vi "禹山电导率校准.vi"() -> ()   [LabVIEW 2016, in "斯坦道多参数.lvlib"]
uses:
  <vilib>/Utility/miscctls.llb/LVPointTypeDef.ctl
  <vilib>/Analysis/NI_AALBase.lvlib
  <vilib>/Analysis/NI_AALPro.lvlib
panel:
  out "滤波设定":dbl
  out "盐度":dbl caption="盐度测量值" format="%#.2f"
  out "通讯状态":string
  out "第二点校准值":dbl
  out "第一点校准值":dbl
  out "最小值":sgl format="%.2g"
  out "最大值":sgl format="%.2g"
  in  "校准停止":bool
  in  "校准模式":u16(ring) items=["两点校准", "单点校准"]
  in  "标液2":dbl
  in  "标液1":dbl
  out "波形图表":sgl(graph) caption="历史曲线"
  out "温度测量值":dbl caption="温度" format="%#.2f"
  out "变异系数":dbl format="%.6g"
  out "standard deviation":dbl caption="标准差" format="%0.2f"
  out "mean":dbl caption="均值" format="%0.2f"
  out "提示":string
  in  "校准启动":bool
  out "测试值":dbl format="%#.2f"
  out "电极斜率":dbl format="%#.6f"
  out "电极零点":dbl format="%#.6f"
  # "电导率电极设定"
  # "℃"
  # "μS/cm"
  # "ppt"
  # "请选择校准模式:"
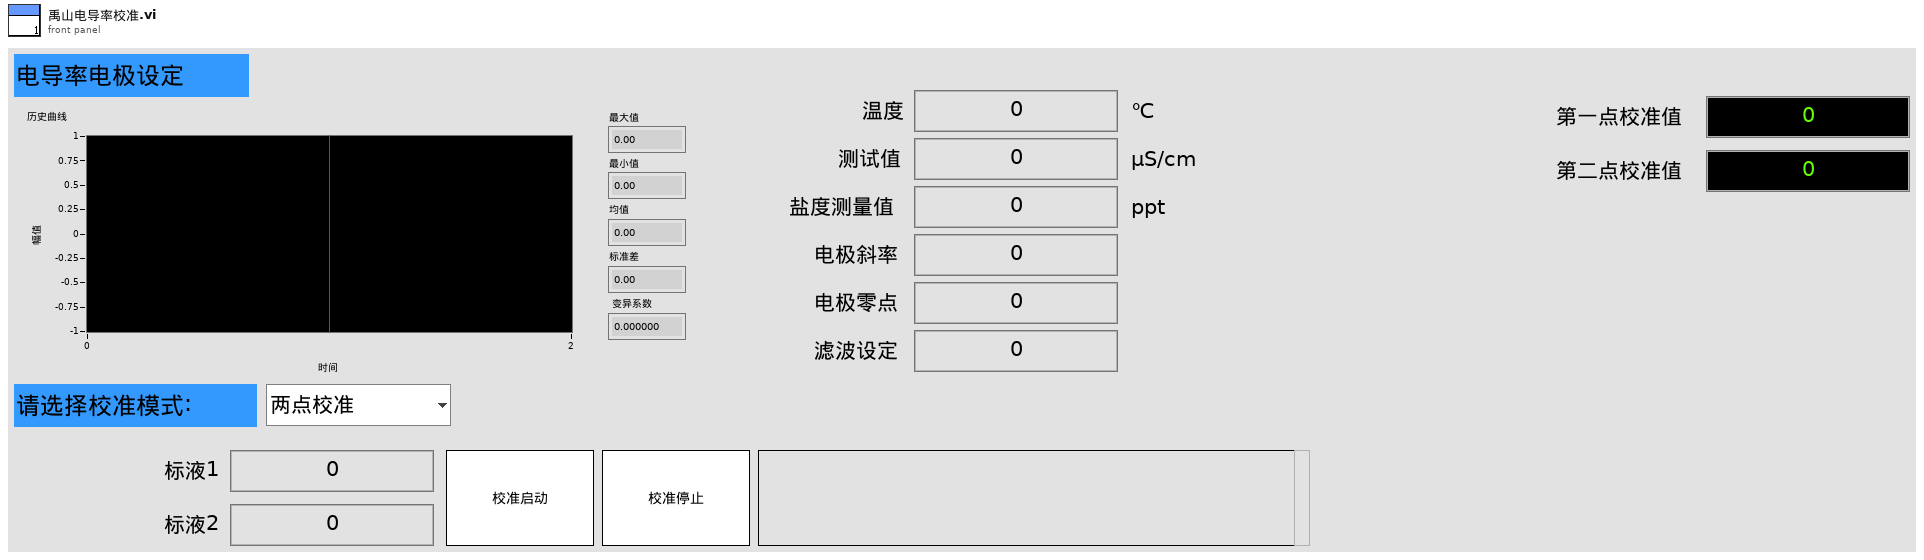
[diagram p1: front panel]
types:
  T1 = typedef "斯坦道多参数.lvlib/通知队列类型.ctl" = enum16{"pH", "DO", "DO2", "Cond", "Turb", "ORP", "叶绿素a", "藻密度", "COD"}
  T2 = typedef "LVPointTypeDef.ctl" = cluster{"Horizontal":i16, "Vertical":i16}
  T3 = cluster{"pH":u32, "DO":u32, "Cond":u32, "Turb":u32, "叶绿素a":u32, "藻密度":u32, "ORP":u32, "COD":u32}
  T4 = cluster{"温度测量值":sgl, "测量值":sgl, "温度偏移修正值":sgl, "信号值":sgl, "数据标识":string}
  T5 = enum8{"Enabled", "Disabled", "Disabled and Grayed Out"}
  T6 = cluster{"ph":bool, "DO":bool, "Cond":bool, "Turb":bool, "叶绿素a":bool, "藻密度":bool, "ORP":bool, "COD":bool, "DO2":bool}
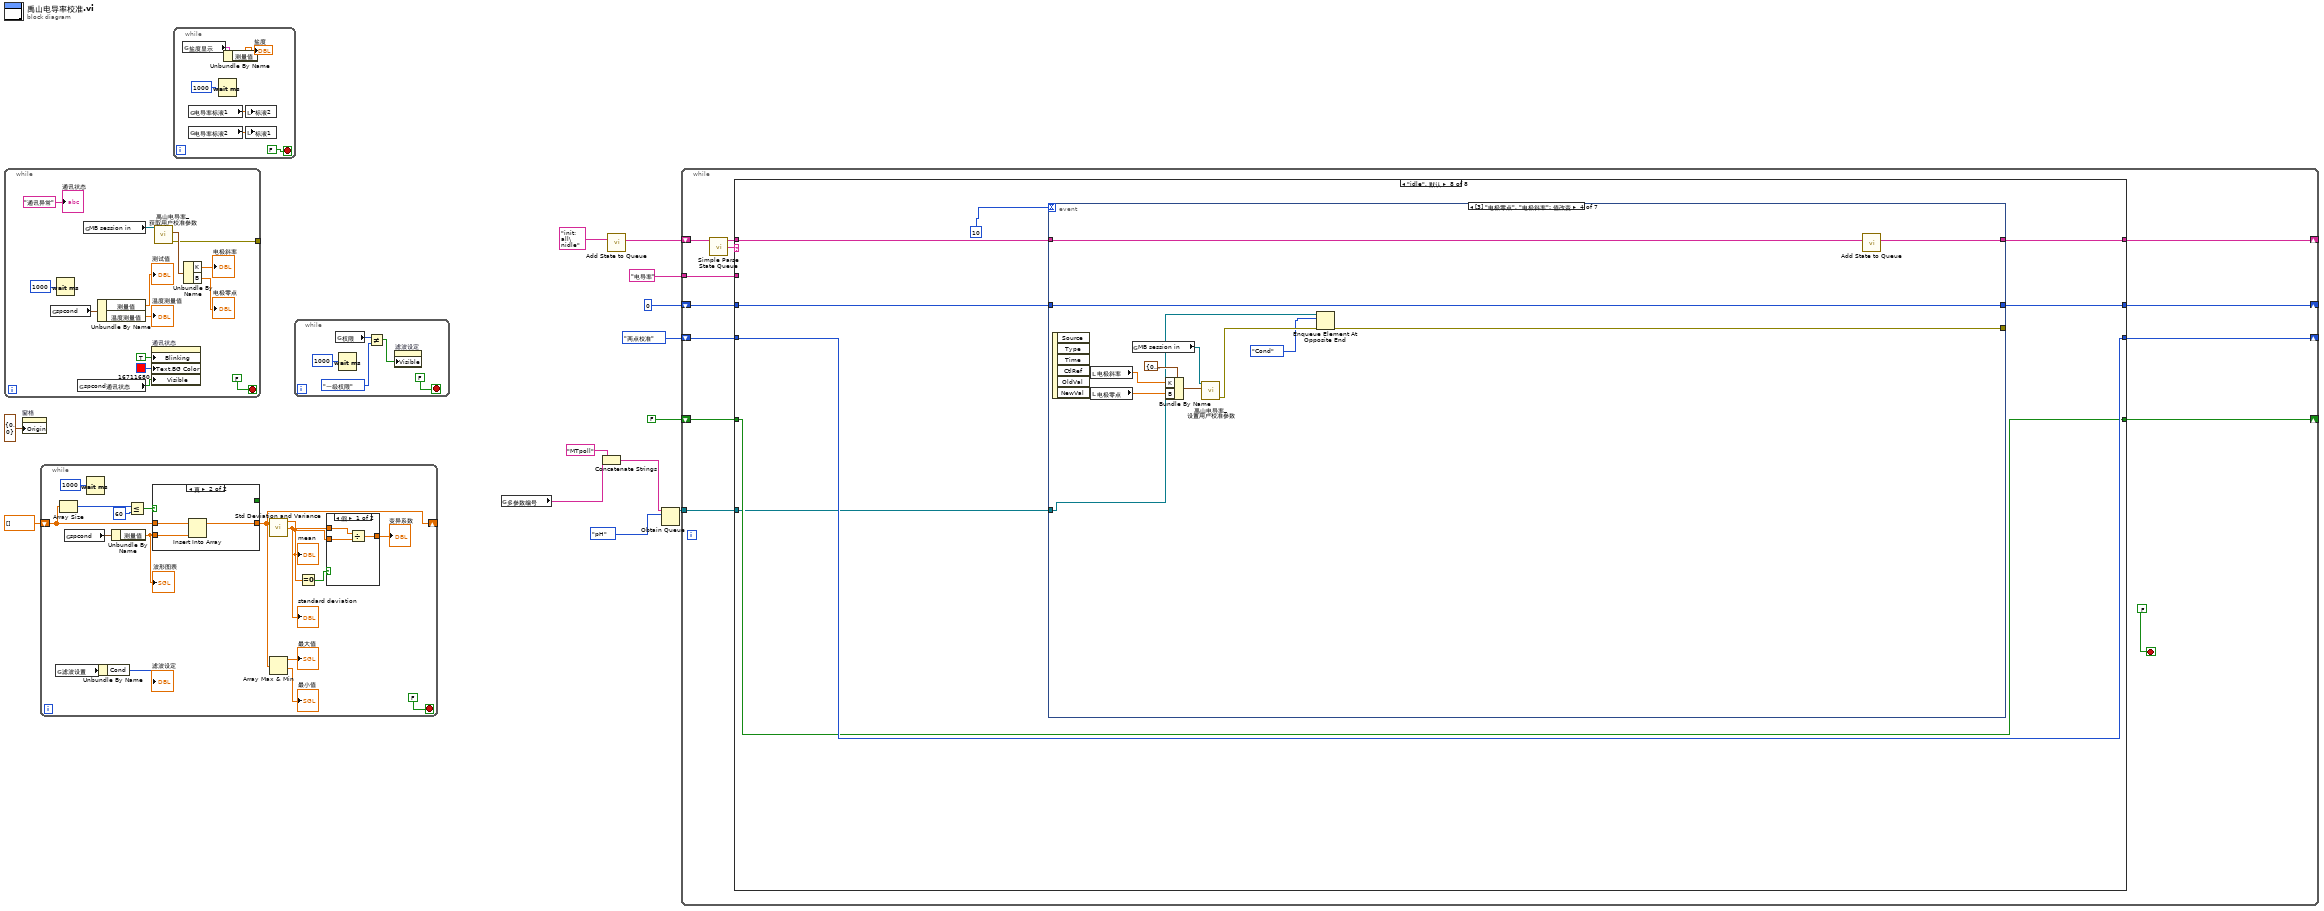
[diagram p0: block diagram]
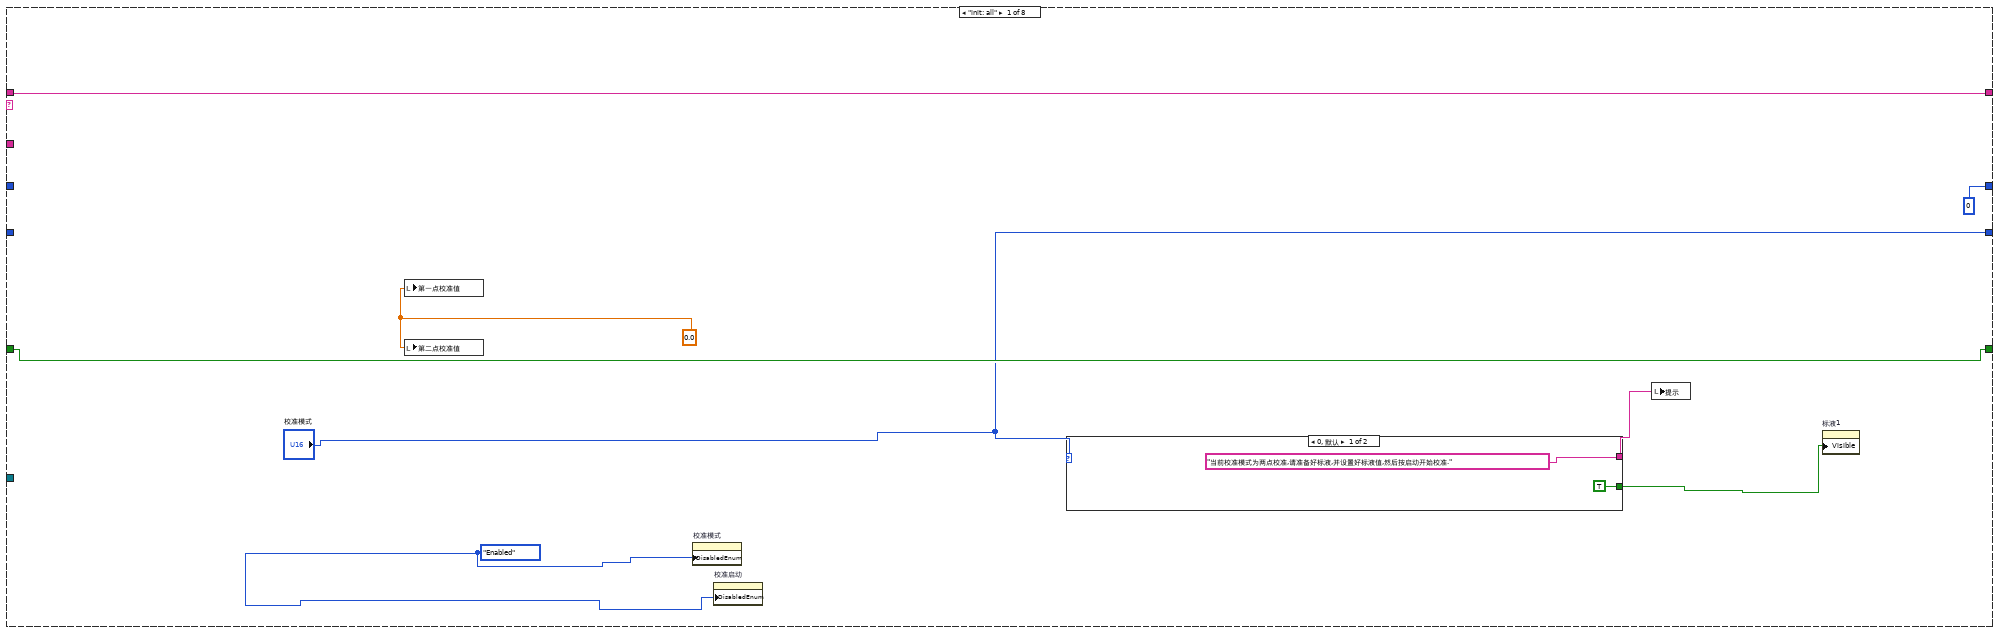
[diagram p2: hidden frame]
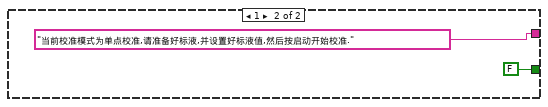
[diagram p3: hidden frame]
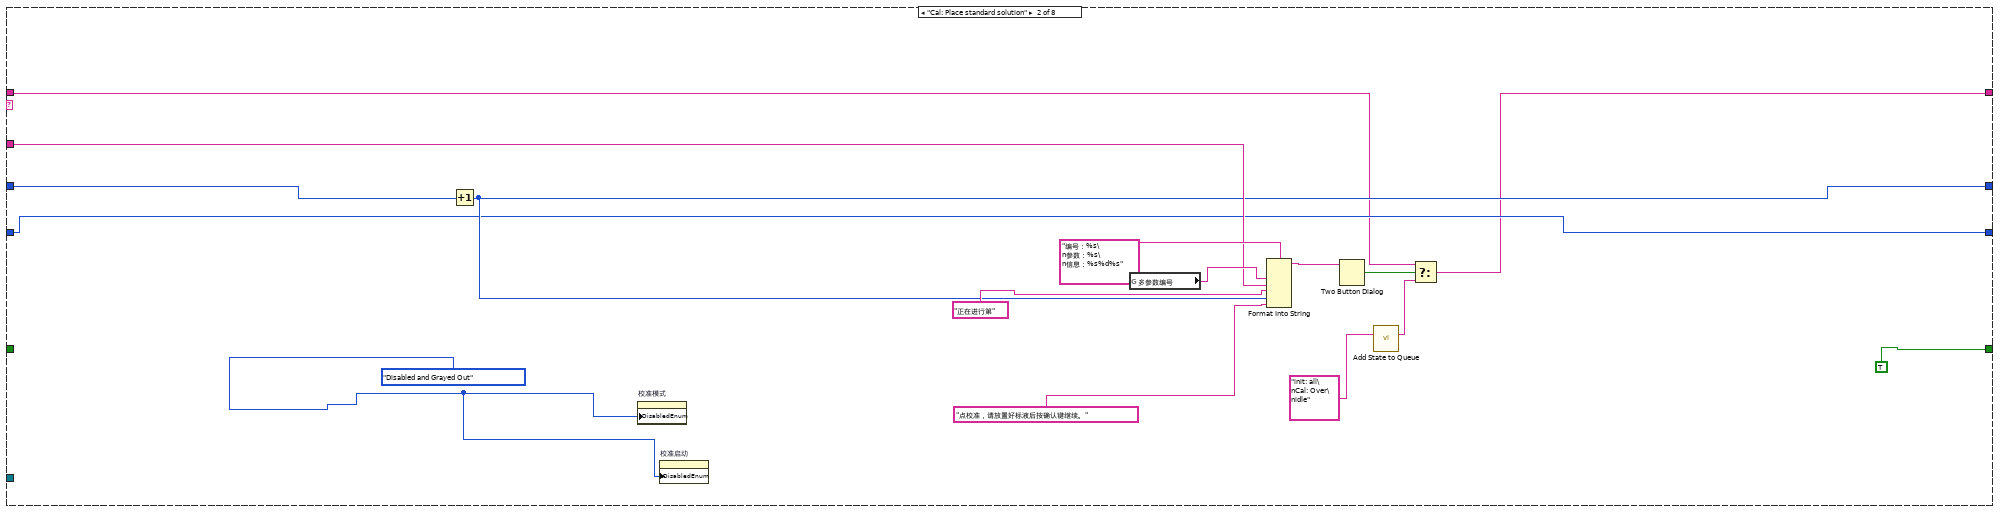
[diagram p4: hidden frame]
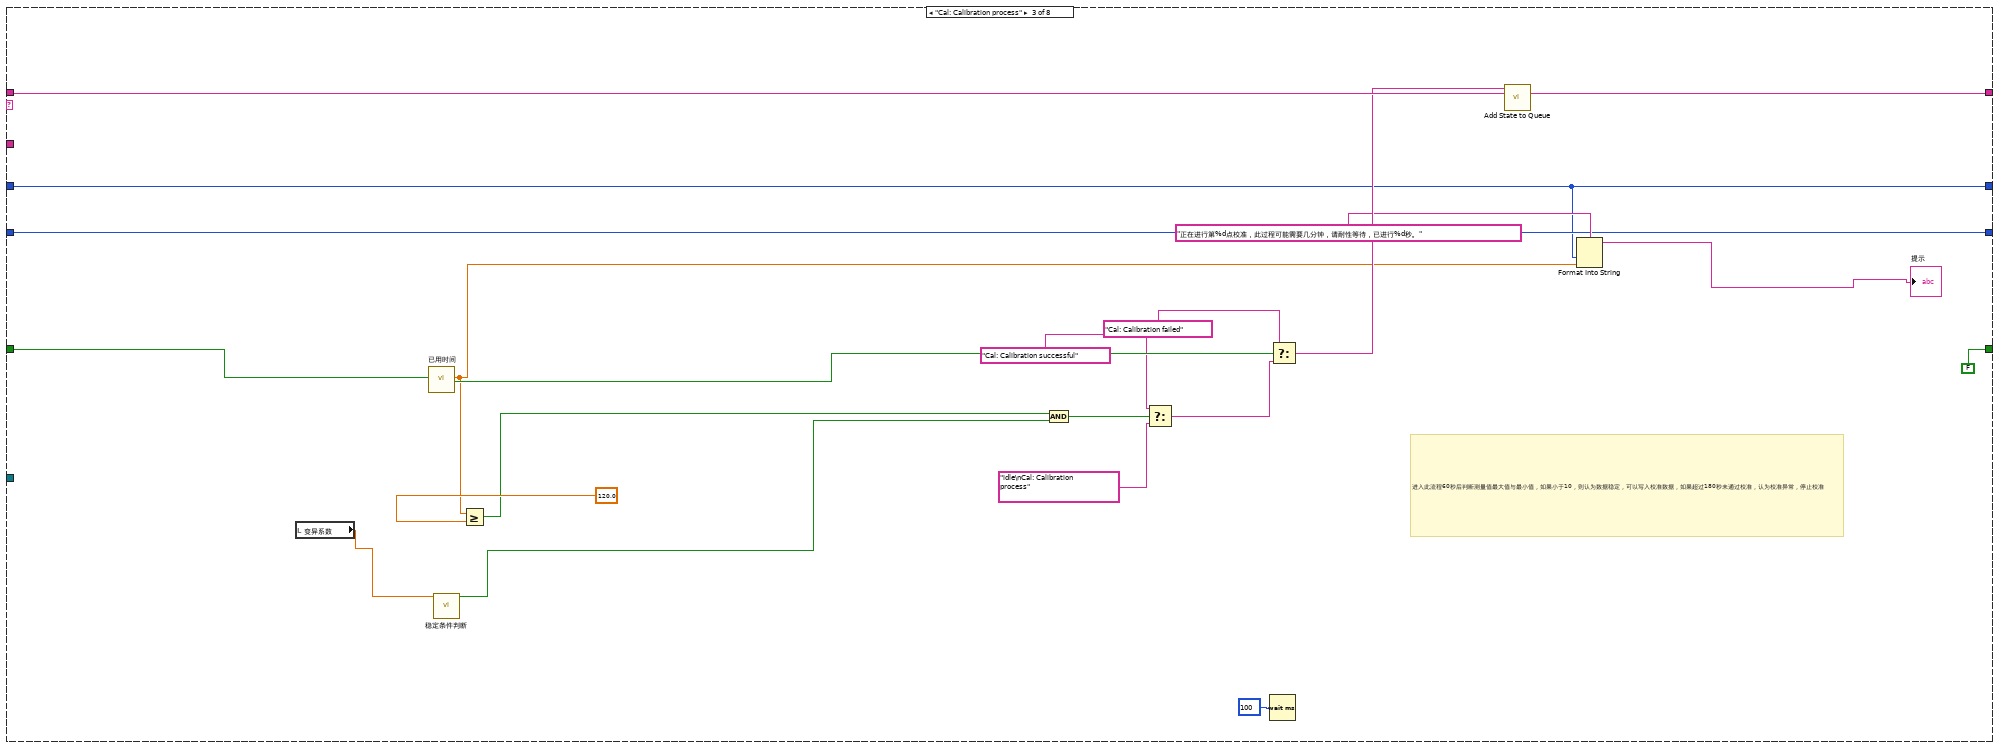
[diagram p5: hidden frame]
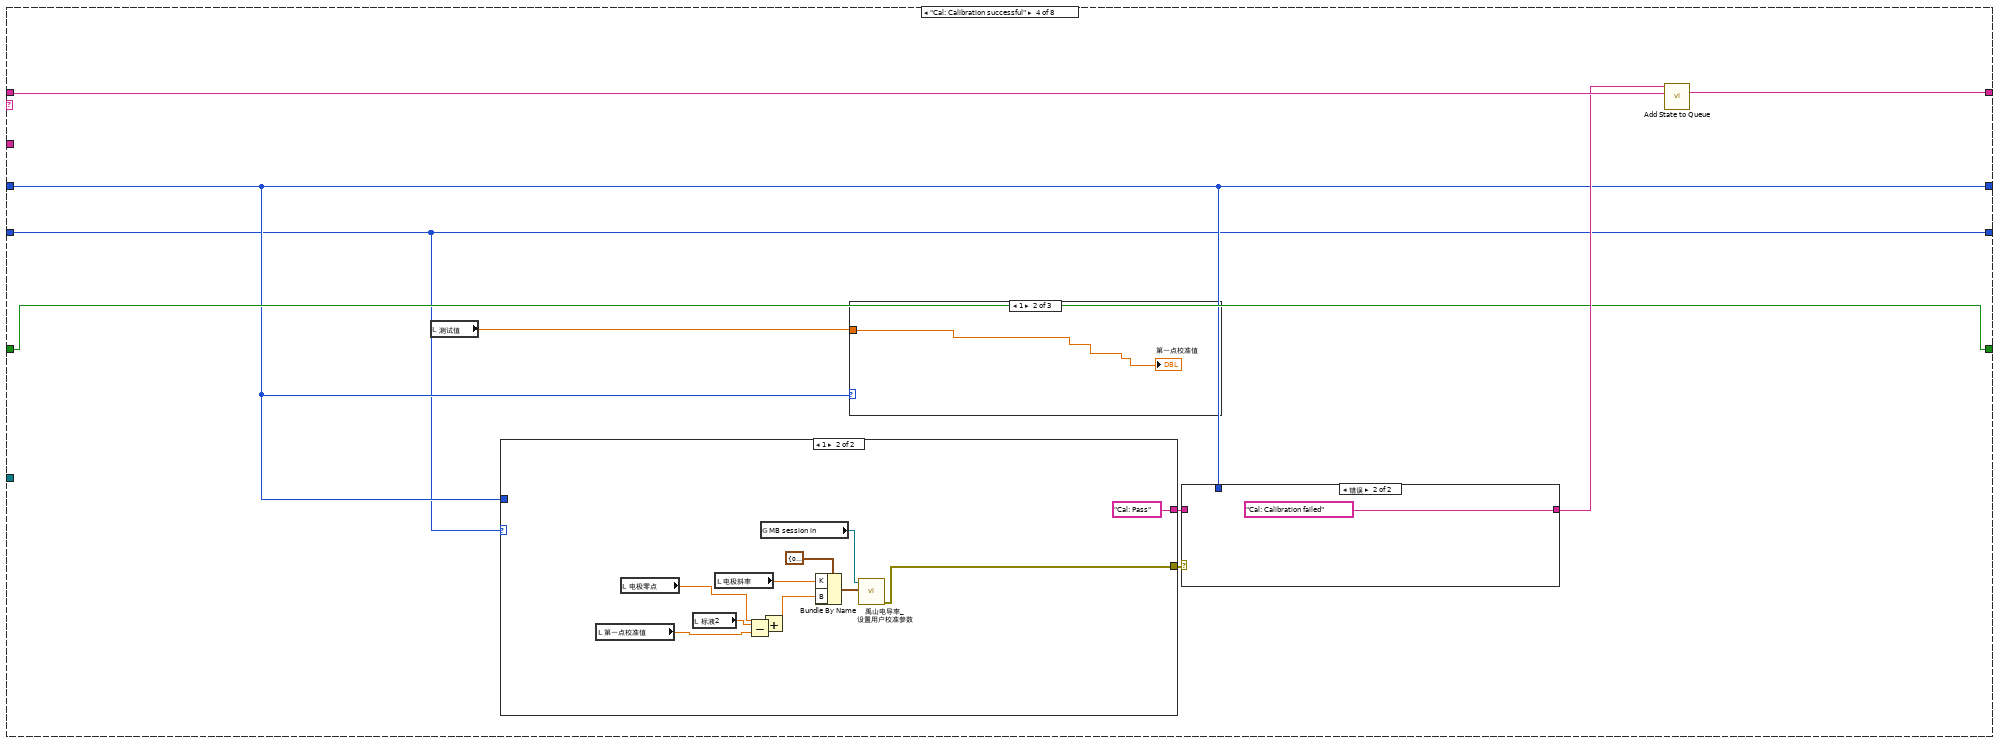
[diagram p6: hidden frame]
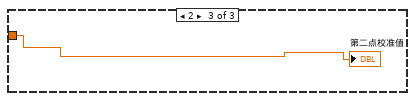
[diagram p8: hidden frame]
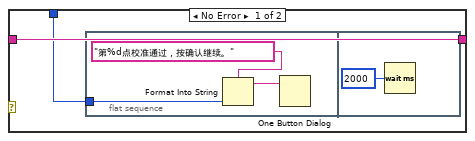
[diagram p9: hidden frame]
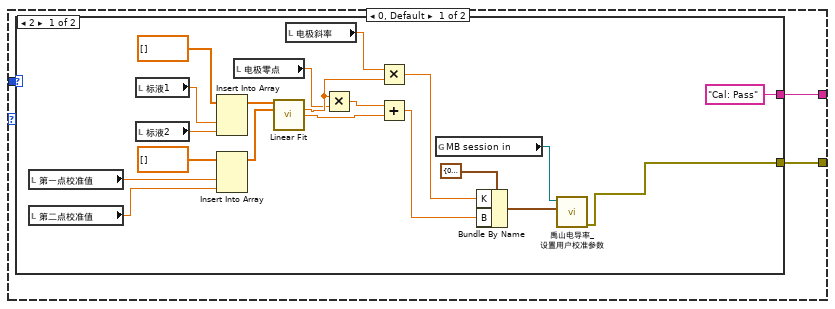
[diagram p10: hidden frame]
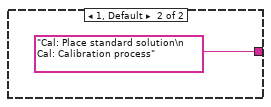
[diagram p11: hidden frame]
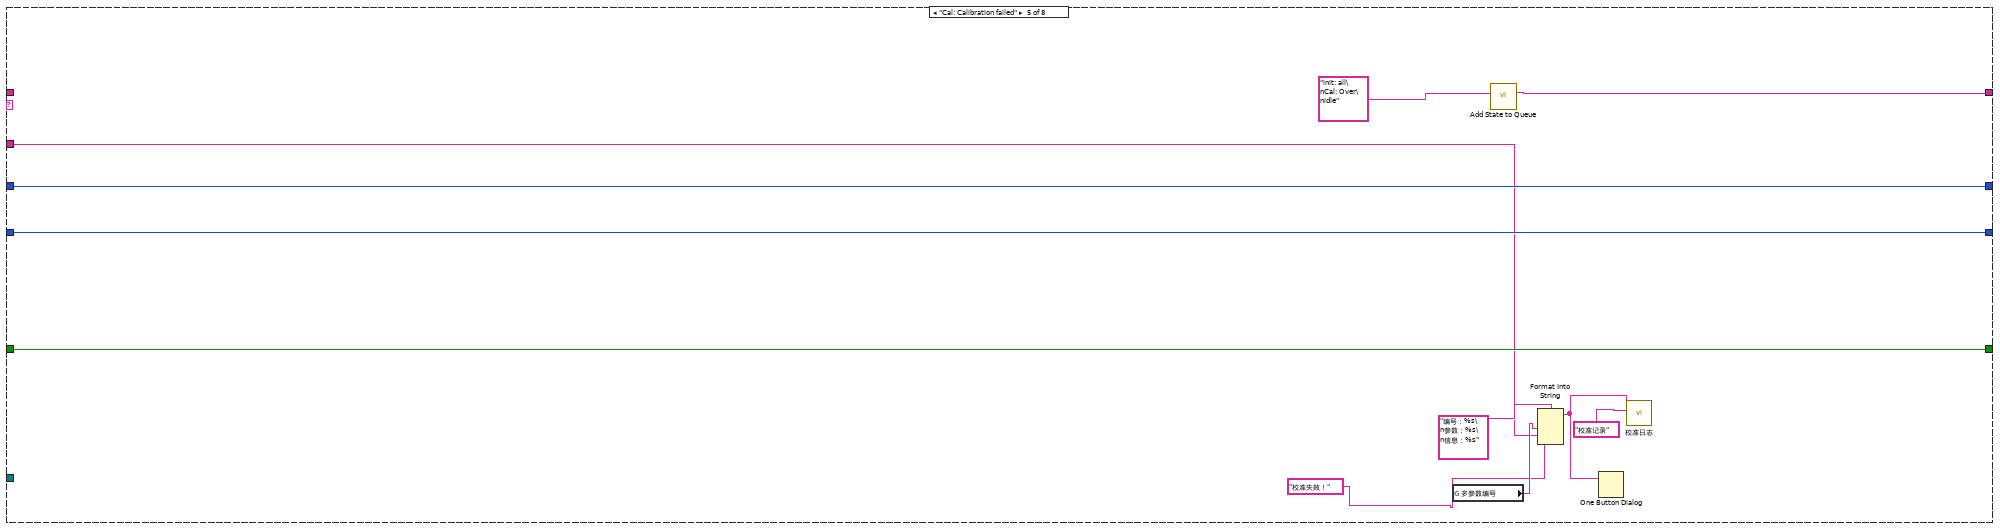
[diagram p12: hidden frame]
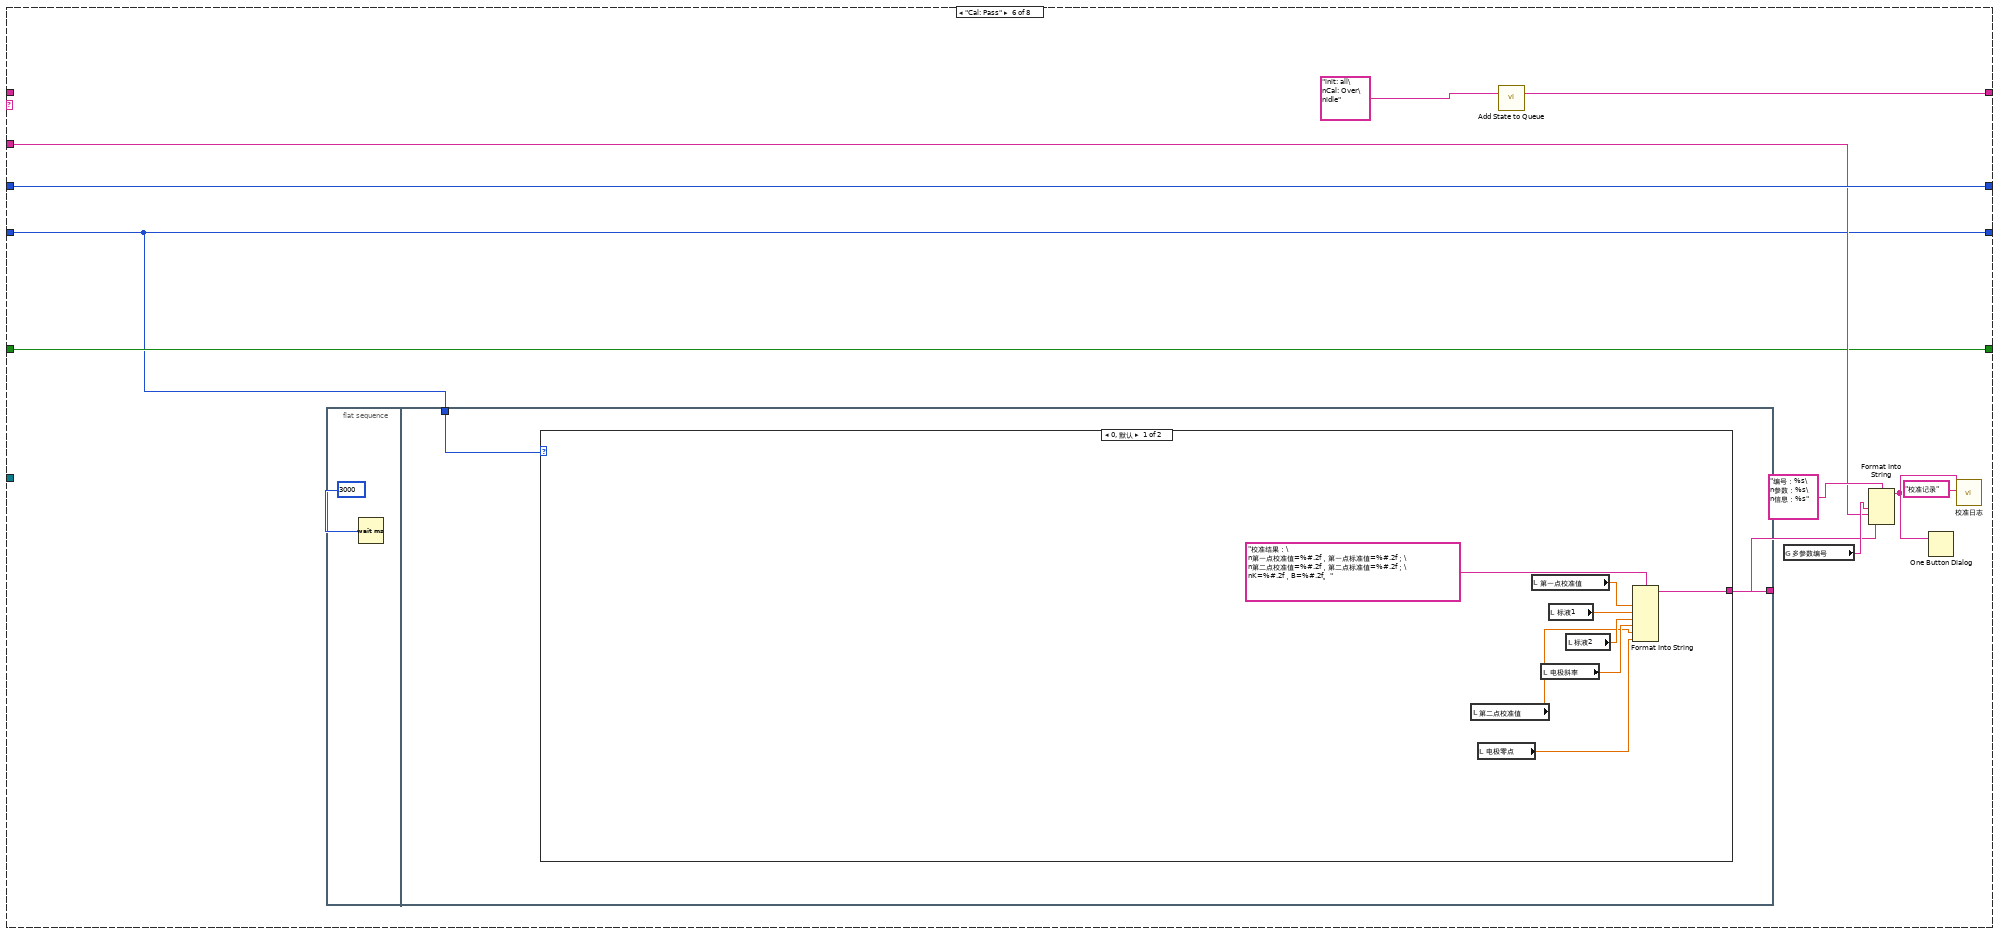
[diagram p13: hidden frame]
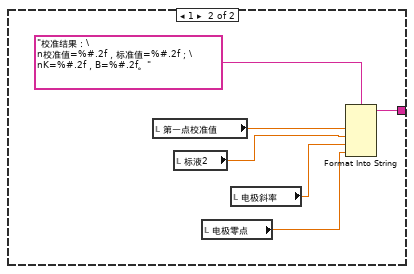
[diagram p14: hidden frame]
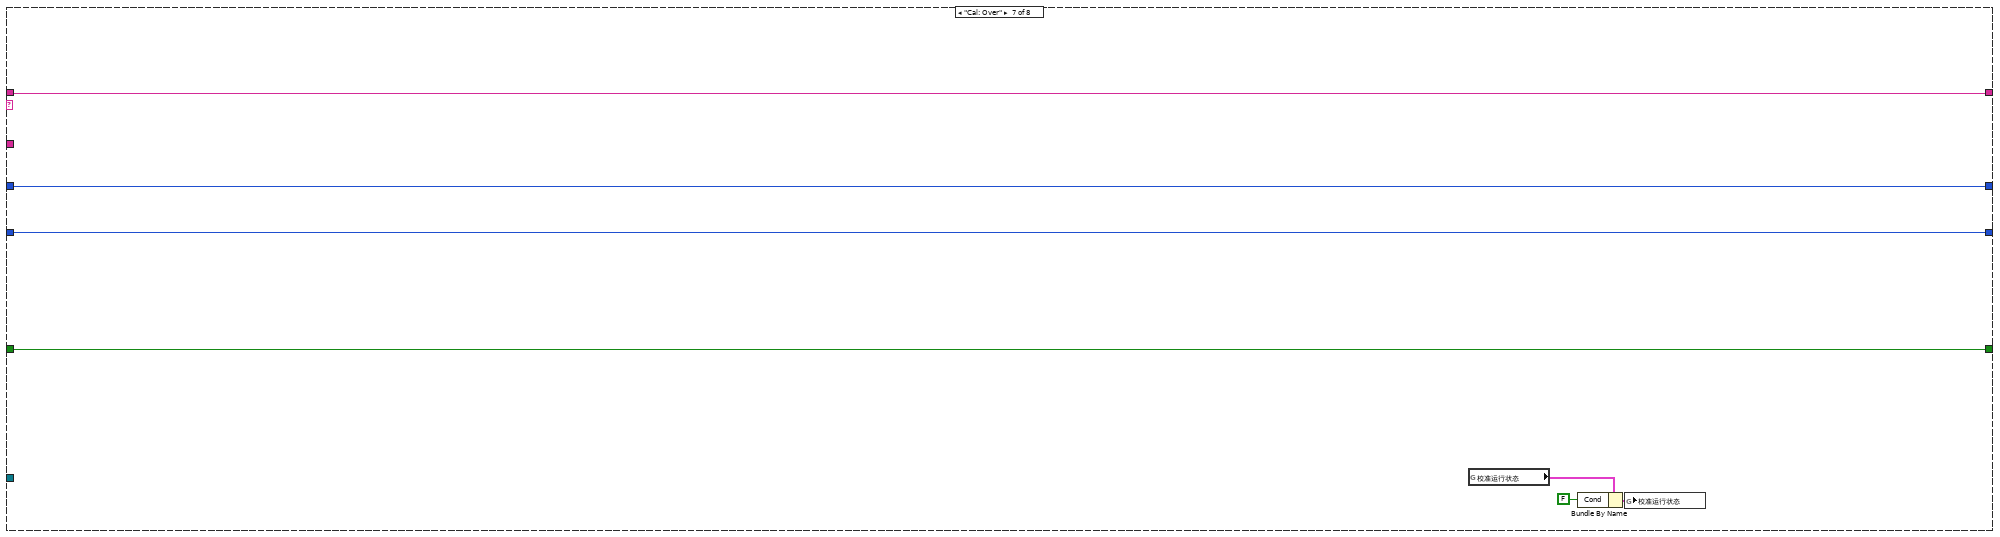
[diagram p15: hidden frame]
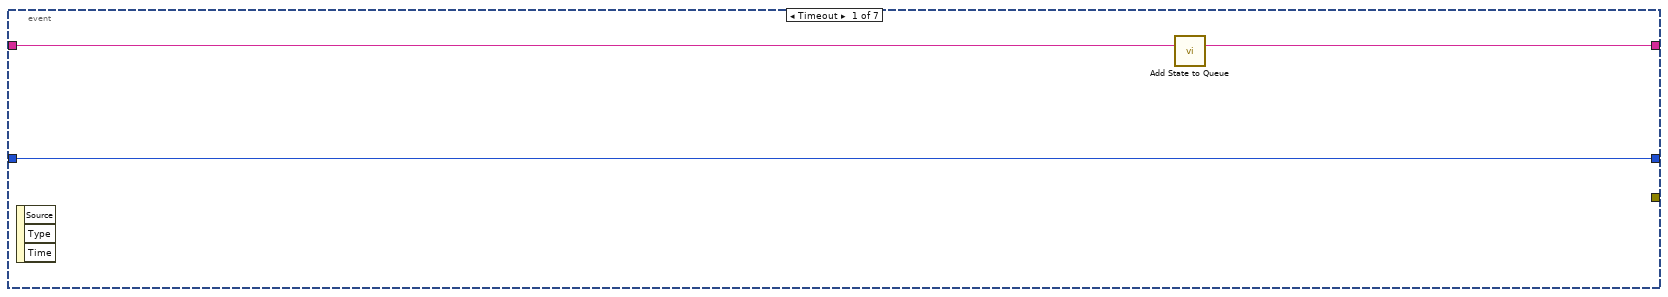
[diagram p16: hidden frame]
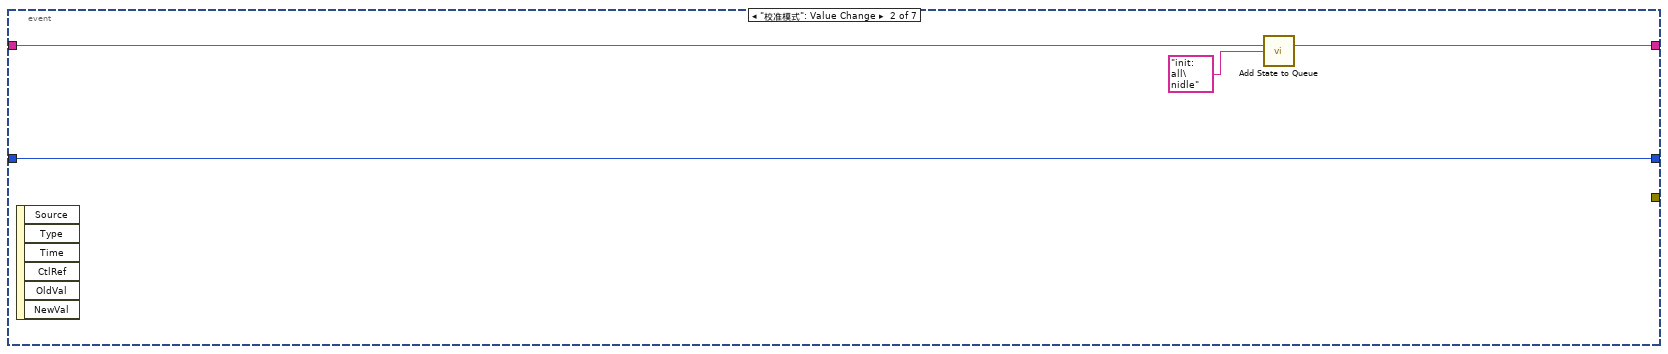
[diagram p17: hidden frame]
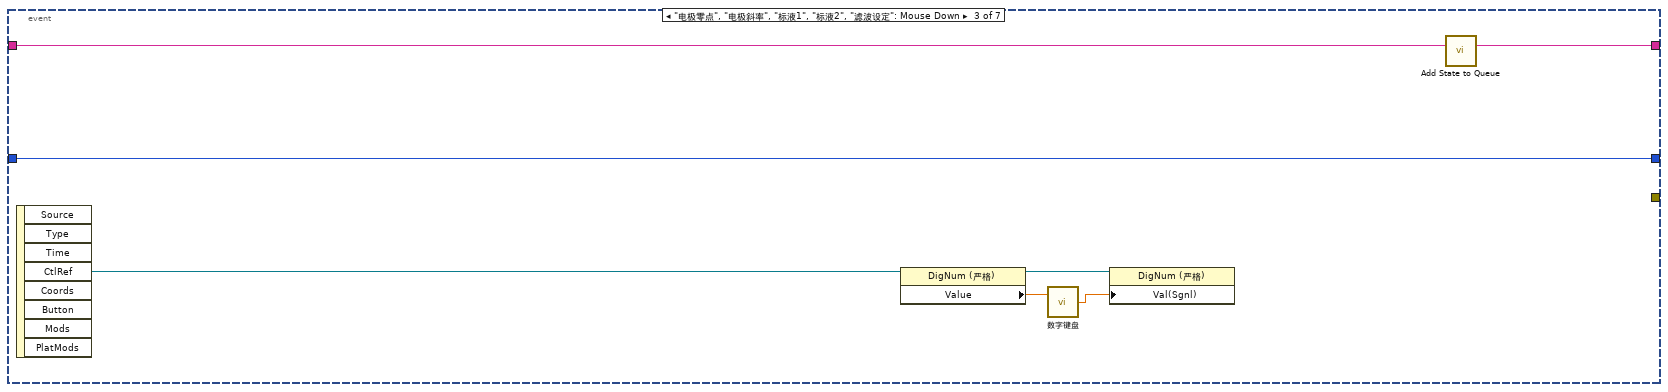
[diagram p18: hidden frame]
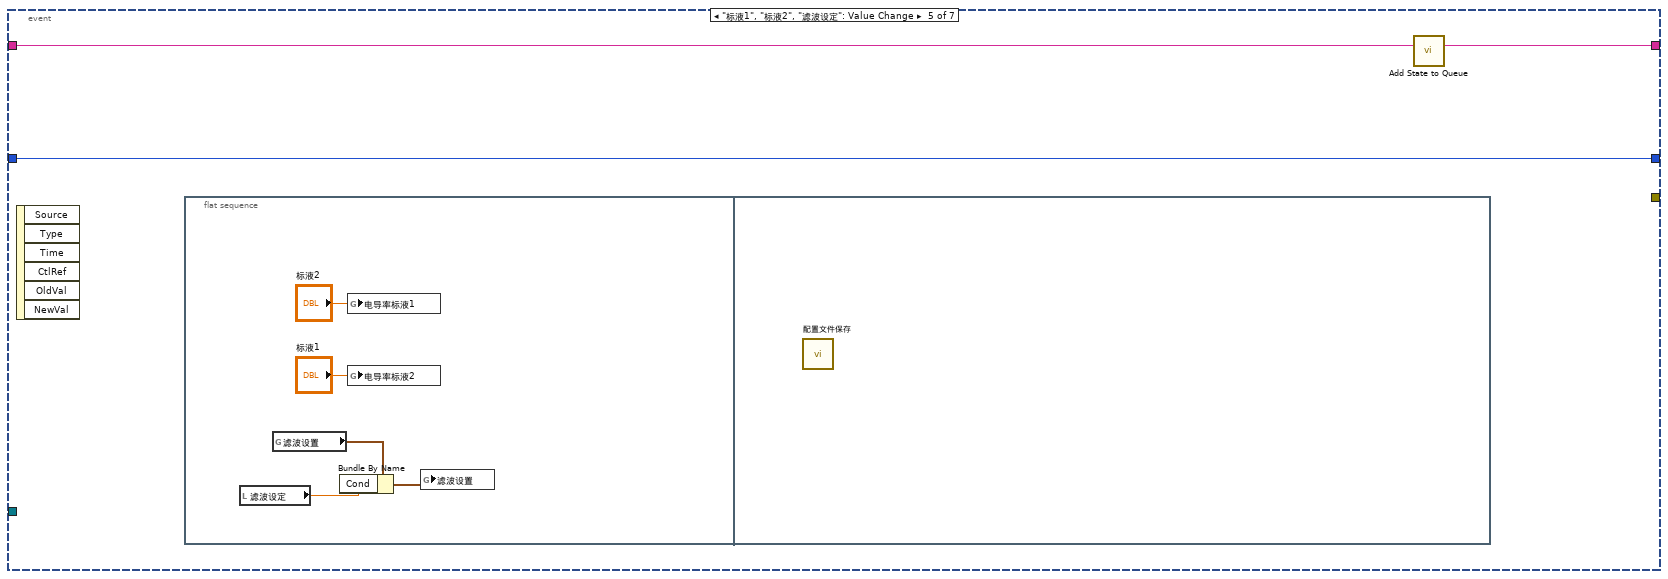
[diagram p19: hidden frame]
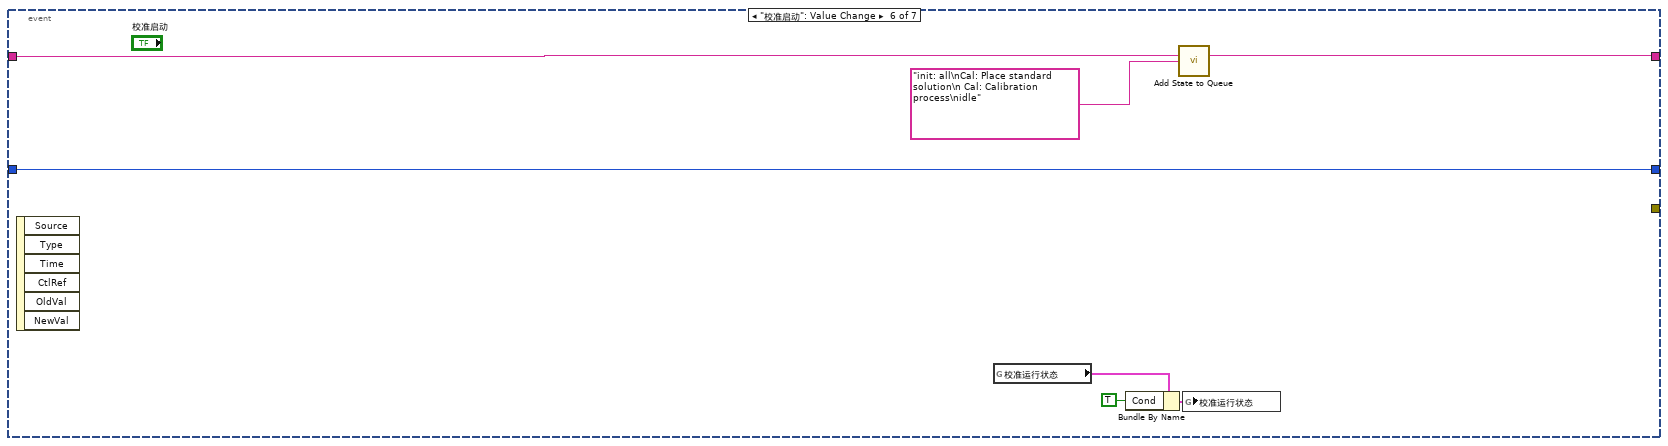
[diagram p20: hidden frame]
diagram:
  n1 = while {
    tunnel: [w22] -> _
    stop <- FALSE stop-if-true
    n2 = global read "禹山过程全局变量.vi" "spcond"() -> (w19:cluster{"温度测量值":sgl, "测量值":sgl, "错误标志":u16})
    n3 = Wait (ms)(milliseconds to wait=u32 1000 ("等待时间（毫秒）")) -> ()  [unwired: 1 out]
    n4 = global read "多参数全局变量.vi" "spcond通讯状态"() -> (w14:bool)
    n5 = global read "多参数全局变量.vi" "MB session in"() -> (w18:refnum<class "MB_Master.lvclass">)
    n6 = Unbundle By Name(w19) -> ("测量值"=→"测试值":sgl, "温度测量值"=→"温度测量值":sgl)
    n7 = property on="通讯状态" class="Str"("Blinking"=TRUE ("闪烁"), "Text.BG Color"=u32 16711680, "Visible"=w14) -> ()  [unwired: 2 in, 2 out]
    n8 = call "禹山电导率_获取用户校准参数.vi"("MB session in"=w18) -> ("error out"=w22:errorcluster, "输出值"=w25:cluster{"K":sgl, "B":sgl})  [unwired: 8 in, 1 out]
    n9 = Unbundle By Name(w25) -> ("K"=→"电极斜率":sgl, "B"=→"电极零点":sgl)
    "通讯状态" <- "通讯异常" ("当前串口")
  }
  n10 = property on="窗格" class="Pane"("Origin"=T2 {"Horizontal"=0, "Vertical"=0} ("原点")) -> ()  [unwired: 2 in, 2 out]
  n11 = while {
    shift-right: [w32] -> _
    shift-left: sgl[] [] -> [w40]
    stop <- FALSE stop-if-true
    n12 = global read "断电保存变量.vi" "滤波设置"() -> (w29:T3)
    n13 = Array Size(array=w40) -> (size(s)=w42:i32)
    n14 = global read "禹山过程全局变量.vi" "spcond"() -> (w34:cluster{"温度测量值":sgl, "测量值":sgl, "错误标志":u16})
    n15 = Wait (ms)(milliseconds to wait=u32 1000 ("等待时间（毫秒）")) -> ()  [unwired: 1 out]
    n16 = Unbundle By Name(w29) -> ("Cond"=→"滤波设定":u32)
    n17 = Unbundle By Name(w34) -> ("测量值"=w33:sgl)
    "波形图表" <- w33
    n18 = Less Or Equal?(x=w42, y=60) -> (x <= y?=w41:bool)
    n19 = case shown="真" w41 {
      tunnel: w40 -> [w53 w56]
      tunnel: w33 -> [w51 w55]
      tunnel: [w49 w54] -> w32
      tunnel: [TRUE _] -> _
      frame False {
        n20 = Replace Array Subset(array=w53, new element=w51) -> (w52:sgl[])  [unwired: 1 in]
        n21 = Rotate 1D Array(1:w52, 2:-1 ("n")) -> (0:w49:sgl[])
      }
      frame True {
        n22 = Insert Into Array(array=w56, new element=w55) -> (w54:sgl[])  [unwired: 1 in]
      }
    }
    n23 = call <vilib>:"Std Deviation and Variance.vi"("X"=w32) -> ("mean"=w35:dbl, "standard deviation"=w36:dbl)  [unwired: 1 in, 1 out]
    "standard deviation" <- w36
    "mean" <- w35
    n24 = Array Max & Min(array=w32) -> (max value=→"最大值":sgl, min value=→"最小值":sgl)  [unwired: 2 out]
    n25 = Equal To 0?(x=w35) -> (x = 0?=w39:bool)
    n26 = case shown="假" w39 {
      tunnel: w36 -> [w47 _]
      tunnel: [w46 _] -> w38
      tunnel: w35 -> [w45 _]
      frame False {
        n27 = Divide(x=w47, y=w45) -> (x/y=w46:dbl)
      }
      frame True {
      }
    }
    "变异系数" <- w38
  }
  n28 = while {
    stop <- FALSE stop-if-true
    n29 = global read "多参数全局变量.vi" "盐度显示"() -> (w58:T4)
    n30 = global read "断电保存变量.vi" "电导率标液1"() -> (w59:dbl)
    n31 = global read "断电保存变量.vi" "电导率标液2"() -> (w60:dbl)
    n32 = Wait (ms)(milliseconds to wait=u32 1000 ("等待时间（毫秒）")) -> ()  [unwired: 1 out]
    n33 = Unbundle By Name(w58) -> ("测量值"=→"盐度":sgl)
    n34 = local write "标液2"(w59) -> ()
    n35 = local write "标液1"(w60) -> ()
  }
  n36 = while {
    stop <- FALSE stop-if-true
    n37 = global read "多参数全局变量.vi" "权限"() -> (w66:enum16{"一级权限", "二级权限", "三级权限"})
    n38 = Wait (ms)(milliseconds to wait=u32 1000 ("等待时间（毫秒）")) -> ()  [unwired: 1 out]
    n39 = Not Equal?(x=w66, y=enum16{"一级权限", "二级权限", "三级权限"}."一级权限") -> (x != y?=w63:bool)
    n40 = property on="滤波设定" class="DigNum (严格)"("Visible"=w63) -> ()  [unwired: 2 in, 2 out]
  }
  n41 = global read "多参数全局变量.vi" "多参数编号"() -> (w3:string)
  n42 = Concatenate Strings("MTpoll" ("名称（未命名）"), w3) -> (w4:string)
  n43 = call "Add State to Queue.vi"("State(s) In (\"\")"="init: all\nidle" ("State(s) In (\"\")")) -> ("States Out"=w10:string)  [unwired: 14 in]
  n44 = Obtain Queue(name (unnamed)=w4, element data type=通知队列类型."pH" ("枚举")) -> (queue out=w2:refnum<queue>)  [unwired: 3 in, 2 out]
  n45 = while {
    shift-right: [w76] -> _
    shift-left: w10 -> [w80]
    shift-right: [w73] -> _
    shift-left: 0 -> [w75]
    tunnel: "电导率" ("State(s) In (\"\")") -> [w74]
    shift-right: [w71] -> _
    shift-left: enum16{"两点校准", "单点校准"}."两点校准" ("校准模式") -> [w72]
    shift-right: [w69] -> _
    shift-left: FALSE -> [w70]
    tunnel: w2 -> [w68]
    stop <- FALSE stop-if-true
    n46 = call "Simple Parse State Queue.vi"("State Queue"=w80) -> ("Remain States"=w77:string, "Next State"=w78:string)  [unwired: 13 in]
    n47 = case shown="\"idle\", 默认" w78 {
      tunnel: w77 -> [w88 w96 w128 w136 _ _ w225 w236]
      tunnel: [w88 w95 w127 w135 w190 w195 w225 w235] -> w76
      tunnel: w75 -> [_ w104 w113 w131 w193 w204 w224 w233]
      tunnel: w74 -> [_ w105 _ _ w184 w200 _ _]
      tunnel: [0 w102 w113 w131 w193 w204 w224 w234] -> w73
      tunnel: w72 -> [_ w101 w114 w130 w192 w196 w223 w232]
      tunnel: ["校准模式" w101 w114 w130 w192 w196 w223 w232] -> w71
      tunnel: w70 -> [w85 _ w116 w132 w191 w199 w222 w230]
      tunnel: [w85 TRUE FALSE w132 w191 w199 w222 w230] -> w69
      tunnel: w68 -> [_ _ _ _ _ _ _ w229]
      frame "init: all" {
        w82 = T5."Enabled" ("禁用")
        w84 = 0.0 ("第一点校准值")
        n48 = local write "第一点校准值"(w84) -> ()
        n49 = local write "第二点校准值"(w84) -> ()
        n50 = property on="校准模式" class="Ring (严格)"("DisabledEnum"=w82) -> ()  [unwired: 2 in, 2 out]
        n51 = property on="校准启动" class="Bool"("DisabledEnum"=w82) -> ()  [unwired: 2 in, 2 out]
        n52 = case shown="0, 默认" "校准模式" {
          tunnel: ["当前校准模式为两点校准,请准备好标液,并设置好标液值,然后按启动开始校准." ("提示") "当前校准模式为单点校准,请准备好标液,并设置好标液值,然后按启动开始校准." ("提示")] -> w87
          tunnel: [TRUE ("可见") FALSE ("可见")] -> w81
          frame 0, Default {
          }
          frame 1 {
          }
        }
        n53 = local write "提示"(w87) -> ()
        n54 = property on="标液1" class="DigNum (严格)"("Visible"=w81) -> ()  [unwired: 2 in, 2 out]
      }
      frame "Cal: Place standard solution" {
        w94 = T5."Disabled and Grayed Out" ("禁用")
        n55 = Increment(x=w104) -> (x+1=w102:i32)
        n56 = property on="校准模式" class="Ring (严格)"("DisabledEnum"=w94) -> ()  [unwired: 2 in, 2 out]
        n57 = property on="校准启动" class="Bool"("DisabledEnum"=w94) -> ()  [unwired: 2 in, 2 out]
        n58 = global read "多参数全局变量.vi" "多参数编号"() -> (w107:string)
        n59 = Format Into String(format string="编号：%s\n参数：%s\n信息：%s%d%s" ("格式字符串"), w107, w105, "正在进行第" ("消息"), w102, "点校准，请放置好标液后按确认键继续。" ("消息")) -> (resulting string=w99:string)  [unwired: 2 in, 1 out]
        n60 = Two Button Dialog(message=w99) -> (T button?=w98:bool)  [unwired: 2 in]
        n61 = call "Add State to Queue.vi"("State(s) In (\"\")"="init: all\nCal: Over\nidle" ("State(s) In (\"\")")) -> ("States Out"=w97:string)  [unwired: 14 in]
        n62 = Select(t=w96, s=w98, f=w97) -> (s? t:f=w95:string)
      }
      frame "Cal: Calibration process" {
        # "进入此流程60秒后判断测量值最大值与最小值，如果小于10，则认为数据稳定，可以写入校准数据，如果超过180秒未通过校准，认为校准异常，停止校准"
        n63 = local read "变异系数"() -> (w110:dbl)
        n64 = call "已用时间"("Reset"=w116) -> ("Elapsed Time (s)"=w112:dbl, "Time has Elapsed"=w129:bool)  [unwired: 11 in, 6 out]
        n65 = call "稳定条件判断.vi"("变异系数"=w110) -> ("布尔"=w109:bool)  [unwired: 10 in]
        n66 = Greater Or Equal?(x=w112, y=120.0) -> (x >= y?=w124:bool)
        n67 = And(x=w124, y=w109) -> (x .and. y?=w121:bool)
        n68 = Select(t="Cal: Calibration successful" ("State(s) In (\"\")"), s=w121, f="idle\nCal: Calibration process" ("State(s) In (\"\")")) -> (s? t:f=w120:string)
        n69 = Wait (ms)(milliseconds to wait=u32 100 ("等待时间（毫秒）")) -> ()  [unwired: 1 out]
        n70 = Select(t="Cal: Calibration failed" ("State(s) In (\"\")"), s=w129, f=w120) -> (s? t:f=w119:string)
        n71 = call "Add State to Queue.vi"("State(s) In Front (\"\")"=w119, "State(s) In (\"\")"=w128) -> ("States Out"=w127:string)  [unwired: 13 in]
        n72 = Format Into String(format string="正在进行第%d点校准，此过程可能需要几分钟，请耐性等待，已进行%d秒。" ("格式字符串"), w113, w112) -> (resulting string=→"提示":string)  [unwired: 2 in, 1 out]
      }
      frame "Cal: Calibration successful" {
        n73 = local read "测试值"() -> (w133:dbl)
        n74 = case shown="1" w130 {
          tunnel: [w150 w172] -> w138
          tunnel: [w149 "Cal: Pass" ("State(s) In (\"\")")] -> w137
          tunnel: w131 -> [w148 _]
          frame 0, Default {
            n75 = case shown="2" w148 {
              tunnel: [w151 _] -> w150
              tunnel: ["Cal: Pass" ("State(s) In (\"\")") "Cal: Place standard solution\n Cal: Calibration process" ("State(s) In (\"\")")] -> w149
              frame 2 {
                n76 = local read "第一点校准值"() -> (w168:dbl)
                n77 = local read "第二点校准值"() -> (w167:dbl)
                n78 = local read "标液1"() -> (w165:dbl)
                n79 = local read "标液2"() -> (w164:dbl)
                n80 = Insert Into Array(array=dbl[] [] ("Weight"), new element #1=w165, new element #2=w164) -> (w163:dbl[])  [unwired: 1 in]
                n81 = Insert Into Array(array=dbl[] [] ("Weight"), new element #1=w168, new element #2=w167) -> (w162:dbl[])  [unwired: 1 in]
                n82 = local read "电极零点"() -> (w155:dbl)
                n83 = call <vilib>:"Linear Fit.vi"("Y"=w163, "X"=w162) -> ("slope"=w156:dbl, "intercept"=w153:dbl)  [unwired: 9 in, 3 out]
                n84 = local read "电极斜率"() -> (w158:dbl)
                n85 = Multiply(x=w156, y=w155) -> (x*y=w154:dbl)
                n86 = Multiply(x=w158, y=w156) -> (x*y=w157:dbl)
                n87 = Add(x=w154, y=w153) -> (x+y=w152:dbl)
                n88 = global read "多参数全局变量.vi" "MB session in"() -> (w161:refnum<class "MB_Master.lvclass">)
                n89 = Bundle By Name(cluster=cluster{"K":sgl, "B":sgl} {"K"=0.0, "B"=0.0} ("用户校准参数"), "K"=w157, "B"=w152) -> (w160:cluster{"K":sgl, "B":sgl})
                n90 = call "禹山电导率_设置用户校准参数.vi"("用户校准参数"=w160, "MB session in"=w161) -> ("error out"=w151:errorcluster)  [unwired: 8 in, 1 out]
              }
              frame 1, Default {
              }
            }
          }
          frame 1 {
            n91 = local read "第一点校准值"() -> (w177:dbl)
            n92 = local read "电极零点"() -> (w173:dbl)
            n93 = local read "标液2"() -> (w176:dbl)
            n94 = local read "电极斜率"() -> (w178:dbl)
            n95 = Subtract(x=w176, y=w177) -> (x-y=w175:dbl)
            n96 = global read "多参数全局变量.vi" "MB session in"() -> (w181:refnum<class "MB_Master.lvclass">)
            n97 = Add(x=w173, y=w175) -> (x+y=w174:dbl)
            n98 = Bundle By Name(cluster=cluster{"K":sgl, "B":sgl} {"K"=0.0, "B"=0.0} ("用户校准参数"), "K"=w178, "B"=w174) -> (w180:cluster{"K":sgl, "B":sgl})
            n99 = call "禹山电导率_设置用户校准参数.vi"("用户校准参数"=w180, "MB session in"=w181) -> ("error out"=w172:errorcluster)  [unwired: 8 in, 1 out]
          }
        }
        n100 = case shown="1" w131 {
          tunnel: w133 -> [_ w139 w140]
          frame 0, Default {
          }
          frame 1 {
            "第一点校准值" <- w139
          }
          frame 2 {
            "第二点校准值" <- w140
          }
        }
        n101 = case shown="错误" w138 {
          tunnel: w137 -> [w142 _]
          tunnel: [w142 "Cal: Calibration failed" ("State(s) In (\"\")")] -> w134
          tunnel: w131 -> [w141 _]
          frame No Error {
            n102 = flat-sequence {
              tunnel: w141 -> [w143]
              frame #0 {
                n103 = Format Into String(format string="第%d点校准通过，按确认继续。" ("格式字符串"), w143) -> (resulting string=w145:string)  [unwired: 2 in, 1 out]
                n104 = One Button Dialog(message=w145) -> ()  [unwired: 1 in, 1 out]
              }
              frame #1 {
                n105 = Wait (ms)(milliseconds to wait=u32 2000 ("等待时间（毫秒）")) -> ()  [unwired: 1 out]
              }
            }
          }
          frame Error {
          }
        }
        n106 = call "Add State to Queue.vi"("State(s) In Front (\"\")"=w134, "State(s) In (\"\")"=w136) -> ("States Out"=w135:string)  [unwired: 13 in]
      }
      frame "Cal: Calibration failed" {
        n107 = global read "多参数全局变量.vi" "多参数编号"() -> (w187:string)
        n108 = call "Add State to Queue.vi"("State(s) In (\"\")"="init: all\nCal: Over\nidle" ("State(s) In (\"\")")) -> ("States Out"=w190:string)  [unwired: 14 in]
        n109 = Format Into String(format string="编号：%s\n参数：%s\n信息：%s" ("格式字符串"), w187, w184, "校准失败！" ("消息")) -> (resulting string=w186:string)  [unwired: 2 in, 1 out]
        n110 = One Button Dialog(message=w186) -> ()  [unwired: 1 in, 1 out]
        n111 = call "校准日志.vi"("table"="校准记录", "日志信息"=w186) -> ()  [unwired: 9 in, 1 out]
      }
      frame "Cal: Pass" {
        n112 = flat-sequence {
          tunnel: [w207] -> w197
          tunnel: w196 -> [w206]
          frame #0 {
            n113 = Wait (ms)(milliseconds to wait=u32 3000 ("等待时间（毫秒）")) -> ()  [unwired: 1 out]
          }
          frame #1 {
            n114 = case shown="0, 默认" w206 {
              tunnel: [w215 w221] -> w207
              frame 0, Default {
                n115 = local read "第二点校准值"() -> (w209:dbl)
                n116 = local read "电极零点"() -> (w208:dbl)
                n117 = local read "第一点校准值"() -> (w213:dbl)
                n118 = local read "电极斜率"() -> (w210:dbl)
                n119 = local read "标液1"() -> (w214:dbl)
                n120 = local read "标液2"() -> (w211:dbl)
                n121 = Format Into String(format string="校准结果：\n第一点校准值=%#.2f，第一点标准值=%#.2f；\n第二点校准值=%#.2f，第二点标准值=%#.2f；\nK=%#.2f，B=%#.2f。" ("提示"), w213, w214, w211, w210, w209, w208) -> (resulting string=w215:string)  [unwired: 2 in, 1 out]
              }
              frame 1 {
                n122 = local read "第一点校准值"() -> (w220:dbl)
                n123 = local read "标液2"() -> (w218:dbl)
                n124 = local read "电极零点"() -> (w216:dbl)
                n125 = local read "电极斜率"() -> (w217:dbl)
                n126 = Format Into String(format string="校准结果：\n校准值=%#.2f，标准值=%#.2f；\nK=%#.2f，B=%#.2f。" ("提示"), w220, w218, w217, w216) -> (resulting string=w221:string)  [unwired: 2 in, 1 out]
              }
            }
          }
        }
        n127 = call "Add State to Queue.vi"("State(s) In (\"\")"="init: all\nCal: Over\nidle" ("State(s) In (\"\")")) -> ("States Out"=w195:string)  [unwired: 14 in]
        n128 = global read "多参数全局变量.vi" "多参数编号"() -> (w201:string)
        n129 = Format Into String(format string="编号：%s\n参数：%s\n信息：%s" ("格式字符串"), w201, w200, w197) -> (resulting string=w198:string)  [unwired: 2 in, 1 out]
        n130 = One Button Dialog(message=w198) -> ()  [unwired: 1 in, 1 out]
        n131 = call "校准日志.vi"("table"="校准记录", "日志信息"=w198) -> ()  [unwired: 9 in, 1 out]
      }
      frame "Cal: Over" {
        n132 = global read "多参数全局变量.vi" "校准运行状态"() -> (w227:T6)
        n133 = Bundle By Name(cluster=w227, "Cond"=FALSE) -> (w228:T6)
        n134 = global write "多参数全局变量.vi" "校准运行状态"(w228) -> ()
      }
      frame "idle", Default {
        n135 = event shown="[3] \"电极零点\", \"电极斜率\": 值改变" {
          selector: _ -> [_ _ _ _ _ _ _]
          dyn-events: _ -> [_ _ _ _ _ _ _]
          timeout: 10 -> [_ _ _ _ _ _ _]
          tunnel: [_ _ _ w253 _ _ _] -> _
          tunnel: w236 -> [w239 w243 w248 w254 w263 w277 _]
          tunnel: [w238 w242 w249 w261 w264 w276 w279] -> w235
          tunnel: [w237 w240 w250 w262 w265 w274 w280] -> w234
          tunnel: w233 -> [w237 w240 w250 w262 w265 w274 w280]
          tunnel: w229 -> [_ _ _ w252 _ _ _]
          event Timeout {
            n136 = event-data() -> ()  [unwired: 1 in, 3 out]
            n137 = call "Add State to Queue.vi"("State(s) In (\"\")"=w239) -> ("States Out"=w238:string)  [unwired: 14 in]
          }
          event "校准模式": Value Change {
            n138 = event-data() -> ()  [unwired: 1 in, 6 out]
            n139 = call "Add State to Queue.vi"("State(s) In (\"\")"=w243, "State(s) At Back (\"\")"="init: all\nidle" ("State(s) In (\"\")")) -> ("States Out"=w242:string)  [unwired: 13 in]
          }
          event "电极零点", "电极斜率", "标液1", "标液2", "滤波设定": Mouse Down {
            n140 = event-data() -> ("CtlRef"=w247:refnum<vi>)  [unwired: 1 in, 7 out]
            n141 = property class="DigNum (严格)"(reference=w247) -> (reference out=w244:refnum<vi>, "Value"=w245:dbl)  [unwired: 1 in, 1 out]
            n142 = call "数字键盘.vi"("OldNumber"=w245) -> ("NewNumber"=w246:dbl)  [unwired: 1 in]
            n143 = property class="DigNum (严格)"(reference=w244, "Val(Sgnl)"=w246) -> ()  [unwired: 1 in, 2 out]
            n144 = call "Add State to Queue.vi"("State(s) In (\"\")"=w248) -> ("States Out"=w249:string)  [unwired: 14 in]
          }
          event "电极零点", "电极斜率": Value Change {
            n145 = event-data() -> ()  [unwired: 1 in, 6 out]
            n146 = local read "电极斜率"() -> (w258:dbl)
            n147 = local read "电极零点"() -> (w257:dbl)
            n148 = global read "多参数全局变量.vi" "MB session in"() -> (w256:refnum<class "MB_Master.lvclass">)
            n149 = Bundle By Name(cluster=cluster{"K":sgl, "B":sgl} {"K"=0.0, "B"=0.0} ("用户校准参数"), "K"=w258, "B"=w257) -> (w259:cluster{"K":sgl, "B":sgl})
            n150 = call "禹山电导率_设置用户校准参数.vi"("用户校准参数"=w259, "MB session in"=w256) -> ("error out"=w255:errorcluster)  [unwired: 8 in, 1 out]
            n151 = Enqueue Element At Opposite End(queue=w252, element=通知队列类型."Cond" ("枚举"), error in (no error)=w255) -> (error out=w253:errorcluster)  [unwired: 1 in, 2 out]
            n152 = call "Add State to Queue.vi"("State(s) In (\"\")"=w254) -> ("States Out"=w261:string)  [unwired: 14 in]
          }
          event "标液1", "标液2", "滤波设定": Value Change {
            n153 = event-data() -> ()  [unwired: 1 in, 6 out]
            n154 = flat-sequence {
              frame #0 {
                n155 = local read "滤波设定"() -> (w266:dbl)
                n156 = global read "断电保存变量.vi" "滤波设置"() -> (w268:T3)
                n157 = Bundle By Name(cluster=w268, "Cond"=w266) -> (w267:T3)
                n158 = global write "断电保存变量.vi" "电导率标液1"("标液2") -> ()
                n159 = global write "断电保存变量.vi" "电导率标液2"("标液1") -> ()
                n160 = global write "断电保存变量.vi" "滤波设置"(w267) -> ()
              }
              frame #1 {
                n161 = call "配置文件保存.vi"() -> ()  [unwired: 12 in]
              }
            }
            n162 = call "Add State to Queue.vi"("State(s) In (\"\")"=w263) -> ("States Out"=w264:string)  [unwired: 14 in]
          }
          event "校准启动": Value Change {
            n163 = event-data() -> ()  [unwired: 1 in, 6 out]
            n164 = global read "多参数全局变量.vi" "校准运行状态"() -> (w272:T6)
            n165 = Bundle By Name(cluster=w272, "Cond"=TRUE) -> (w273:T6)
            n166 = call "Add State to Queue.vi"("State(s) In (\"\")"=w277, "State(s) At Back (\"\")"="init: all\nCal: Place standard solution\n Cal: Calibration process\nidle" ("State(s) In (\"\")")) -> ("States Out"=w276:string)  [unwired: 13 in]
            n167 = global write "多参数全局变量.vi" "校准运行状态"(w273) -> ()
          }
          event "校准停止": Value Change {
            n168 = event-data() -> ()  [unwired: 1 in, 6 out]
            n169 = call "Add State to Queue.vi"("State(s) In (\"\")"="init: all\nCal: Over\nidle" ("State(s) In (\"\")")) -> ("States Out"=w279:string)  [unwired: 14 in]
          }
        }
      }
    }
  }
